vi "SyntaxOperation_Logic.vi"(8 "error in (no error)":errorcluster, 11 "Logical Parsed Expression":T1) -> (0 "error out":errorcluster, 1 "Error Index Out":i32, 2 "Token":string[](array[string]), 3 "Logical Parsed Expression Out":T1)   [LabVIEW 2014, in "SeqLoop.lvlib"]
uses:
  SeqLoop.lvlib
  TypeDefs/LogicParsedExpression.ctl
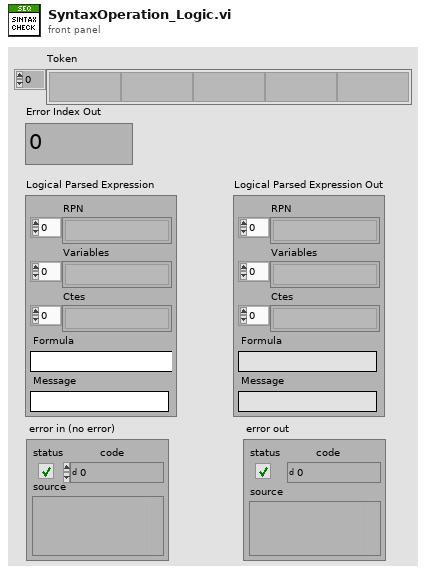
[diagram p1: front panel]
types:
  T1 = typedef "SeqLoop.lvlib/LogicParsedExpression.ctl" = cluster{"RPN ":string[], "Variables":string[], "Ctes":string[], "Formula":string, "Message":string}
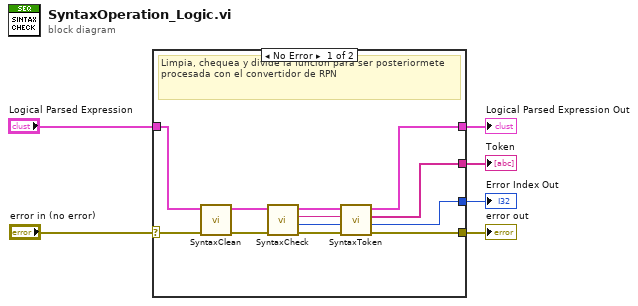
[diagram p0: block diagram]
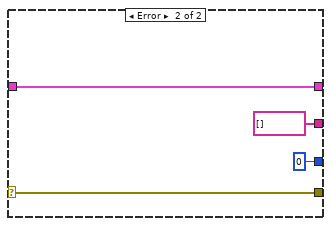
[diagram p2: hidden frame]
diagram:
  n1 = case shown="No Error" "error in (no error)" {
    selector: "error in (no error)" -> [w13 w21]
    tunnel: [w15 w21] -> w6
    tunnel: "Logical Parsed Expression" -> [w14 w22]
    tunnel: [w18 w22] -> w2
    tunnel: [w17 string[] [] ("Token")] -> w4
    tunnel: [w16 0 ("Error Index Out")] -> w3
    frame No Error {
      # "Limpia, chequea y divide la función para ser posteriormete procesada con el convertidor de RPN"
      n2 = call "SyntaxClean.vi"("error in (no error)"=w13, "Logical Parsed Expression"=w14) -> ("error out"=w12:errorcluster, "Logical Parsed Expression Out"=w10:T1)  [unwired: 8 in]
      n3 = call "SyntaxCheck.vi"("error in"=w12, "Logical Parsed Expression"=w10) -> ("error out"=w11:errorcluster, "Error Index"=w7:i32, "Funcion Analizada"=w8:string, "Logical Parsed Expression Out"=w9:T1)  [unwired: 6 in]
      n4 = call "SyntaxToken.vi"("error in"=w11, "Error Index In"=w7, "Funcion Analizada"=w8, "Logical Parsed Expression"=w9) -> ("error out"=w15:errorcluster, "Error Index Out"=w16:i32, "Token"=w17:string[], "Logical Parsed Expression Out"=w18:T1)  [unwired: 4 in]
    }
    frame Error {
    }
  }
  "error out" <- w6
  "Error Index Out" <- w3
  "Token" <- w4
  "Logical Parsed Expression Out" <- w2
